vi "SetSlopeCompensation.vi"(8 "error in":T1, 10 "Z/Y":sgl=-inf format="%#_g %", 11 "Z/X":sgl=-inf format="%#_g %") -> (0 "error out":T1, 2 "Z/Y out":sgl format="%#_g %", 3 "Z/X out":sgl format="%#_g %")   [LabVIEW 2016]
doc: "In both directions ('X' and 'Y') a value between -20% and +20% is accepted. By passing -Inf as input values, the corresponding parameter(s) will be read out."
uses:
  Controls/Error_Out.ctl
  Files_ASC500/DLL/ASC500_RemoteControlV27.dll
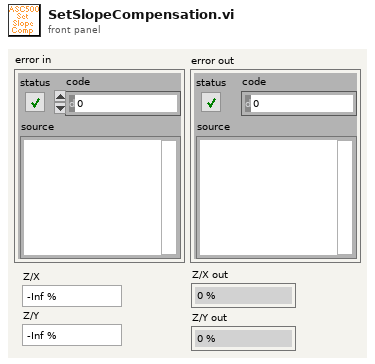
[diagram p1: front panel]
types:
  T1 = typedef "Error_Out.ctl" = errorcluster
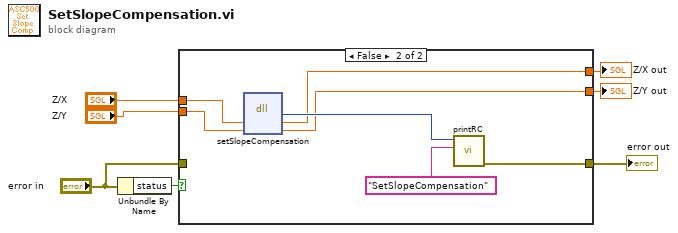
[diagram p0: block diagram]
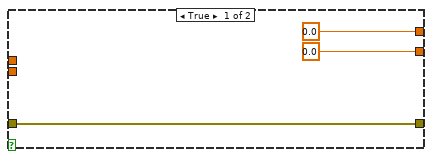
[diagram p2: hidden frame]
diagram:
  n1 = Unbundle By Name("error in") -> ("status"=w6:bool)
  n2 = case shown="False" w6 {
    tunnel: [w10 w17] -> w7
    tunnel: "Z/X" -> [_ w14]
    tunnel: "Z/Y" -> [_ w13]
    tunnel: "error in" -> [w10 _]
    tunnel: [sgl 0.0 ("X") w12] -> w2
    tunnel: [sgl 0.0 ("Y") w11] -> w1
    frame True {
    }
    frame False {
      n3 = dll-call lib="G:/SCMOperations/Share/ELE/Produkt Information/ASC500/04 Remote Control/02 development versions/2018Nov06/Files_ASC500/DLL/ASC500_RemoteControlV27.dll" fn="setSlopeCompensation"("X"=w14, "Y"=w13) -> ("return type"=w16:i32, "X"=w12:sgl, "Y"=w11:sgl)  [unwired: 3 in, 2 out]
      n4 = call "printRC.vi"("additional information"="SetSlopeCompensation", "RC"=w16) -> ("error out"=w17:T1)  [unwired: 9 in]
    }
  }
  "error out" <- w7
  "Z/X out" <- w2
  "Z/Y out" <- w1
